vi "run time calculator.vi"(8 "Volume unit":u16(ring) items=["µL", "nL", "mL"], 9 "Volume":i32=100, 10 "Flow Rate Units (1:ml/min)":u32(ring)=3 items=["ml/hr", "ml/min", "ul/hr", "ul/min", "ul/sec", "nl/sec"], 11 "Flow rate":dbl=2.0) -> (2 "time in seconds":dbl)   [LabVIEW 2016]
panel:
  out "Current flow rate unit":i32
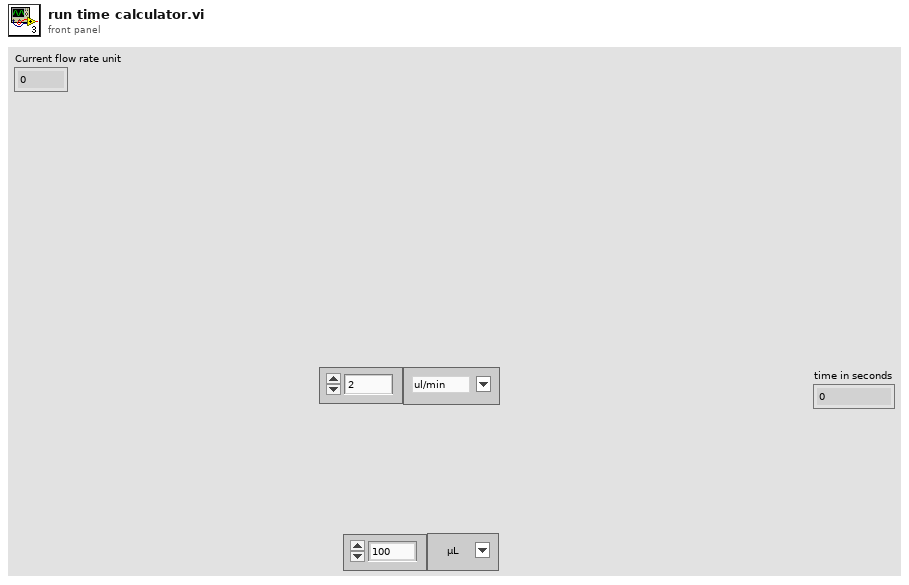
[diagram p1: front panel]
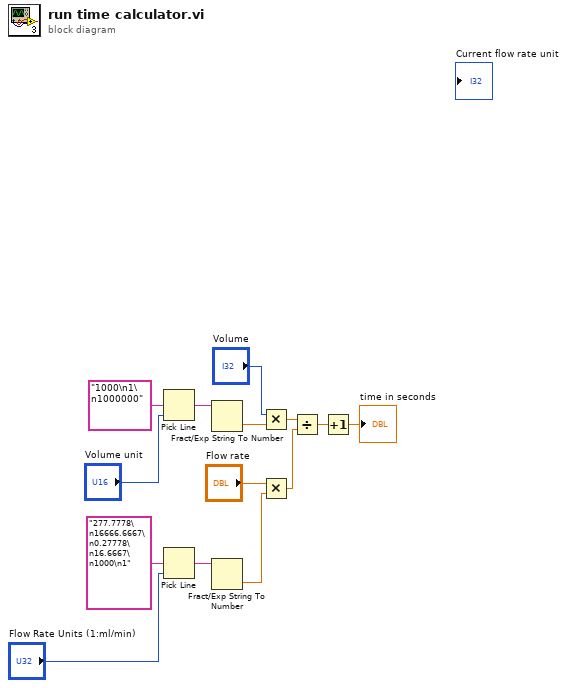
[diagram p0: block diagram]
diagram:
  n1 = Pick Line(multi-line string="1000\n1\n1000000", line index="Volume unit") -> (output string=w6:string)  [unwired: 1 in]
  n2 = Pick Line(multi-line string="277.7778\n16666.6667\n0.27778\n16.6667\n1000\n1", line index="Flow Rate Units (1:ml/min)") -> (output string=w10:string)  [unwired: 1 in]
  n3 = Fract/Exp String To Number(string=w6) -> (number=w5:dbl)  [unwired: 3 in, 1 out]
  n4 = Fract/Exp String To Number(string=w10) -> (number=w8:dbl)  [unwired: 3 in, 1 out]
  n5 = Multiply(x="Volume", y=w5) -> (x*y=w4:dbl)
  n6 = Multiply(x="Flow rate", y=w8) -> (x*y=w3:dbl)
  n7 = Divide(x=w4, y=w3) -> (x/y=w1:dbl)
  n8 = Increment(x=w1) -> (x+1=→"time in seconds":dbl)
